vi "Ejemplo7_Strings.vi"() -> ()   [LabVIEW 2020]
panel:
  out "ACTUADOR 3":string
  out "ACTUADOR 2":string
  out "ACTUADOR 1":string
  in  "Contactor":bool
  in  "Termocupla":dbl(slide) scale=0.0..100.0
  in  "Motor":i16(knob) scale=0.0..60.0
  out "length":i32
  out "Salida":string
  in  "Registrar":bool
  in  "Indique Nombre":string
  in  "Indique Apellido":string
  out "Minusculas":string
  out "Mayusculas":string
  out "Subset":string
  out "String Concatenate":string
  out "N Caracteres":i32
  out "Dato B":string
  in  "Dato A":string
  # "Strings"
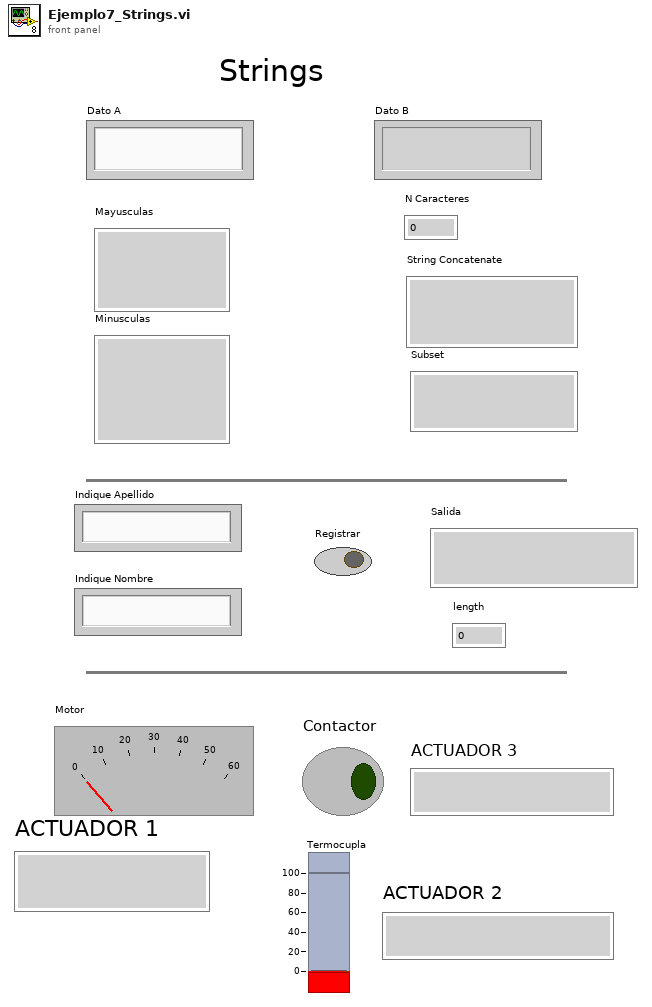
[diagram p1: front panel]
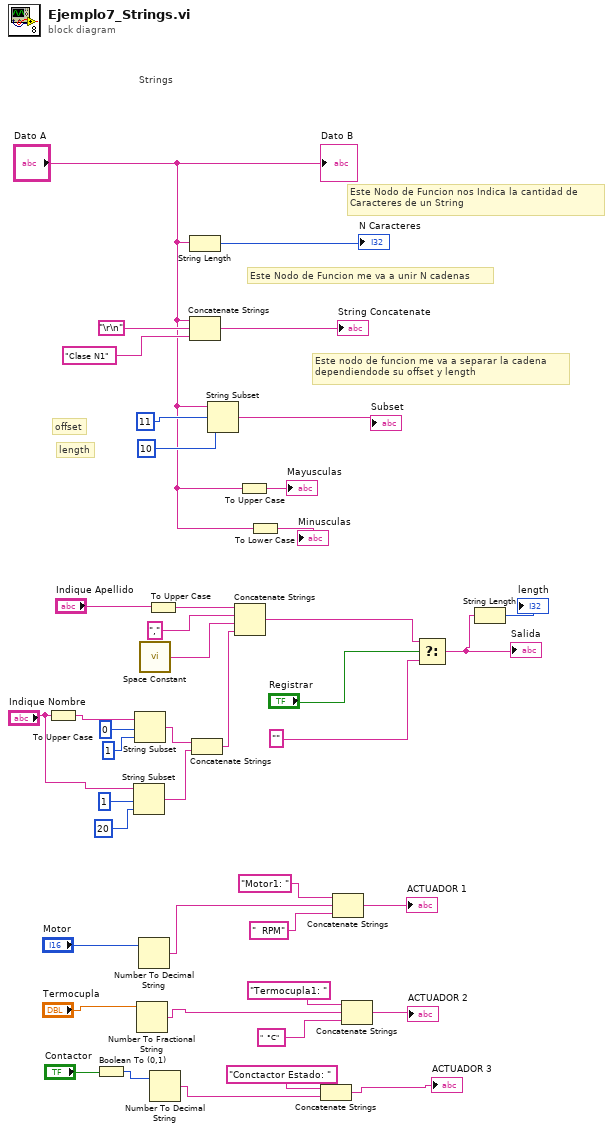
[diagram p0: block diagram]
diagram:
  # "length"
  # "offset"
  # "Este nodo de funcion me va a separar la cadena \ndependiendode su offset y length"
  # "Este Nodo de Funcion me va a unir N cadenas"
  # "Este Nodo de Funcion nos Indica la cantidad de \nCaracteres de un String"
  # "Strings"
  n1 = To Upper Case(1:"Indique Nombre") -> (0:w23:string)
  n2 = Boolean To (0,1)(Boolean="Contactor") -> (0, 1=w4:i16)
  n3 = String Subset(string="Indique Nombre", offset (0)=1 ("length (rest)"), length (rest)=20 ("length (rest)")) -> (substring=w24:string)
  n4 = String Subset(string=w23, offset (0)=0 ("length (rest)"), length (rest)=1 ("length (rest)")) -> (substring=w25:string)
  n5 = Number To Fractional String(number="Termocupla") -> (F-format string=w7:string)  [unwired: 3 in]
  n6 = Number To Decimal String(number="Motor") -> (decimal integer string=w13:string)  [unwired: 1 in]
  n7 = call <vilib>:"Space Constant.vi"() -> ("String"=w30:string)
  n8 = To Upper Case(1:"Indique Apellido") -> (0:w32:string)
  n9 = Number To Decimal String(number=w4) -> (decimal integer string=w2:string)  [unwired: 1 in]
  n10 = String Length(string="Dato A") -> (length=→"N Caracteres":i32)
  n11 = Concatenate Strings("Dato A", "\r\n", "Clase N1") -> (→"String Concatenate":string)
  n12 = Concatenate Strings(w25, w24) -> (w22:string)
  n13 = String Subset(string="Dato A", offset (0)=11, length (rest)=10 ("length (rest)")) -> (substring=→"Subset":string)
  n14 = Concatenate Strings(w32, ",", w30, w22) -> (w20:string)
  n15 = To Upper Case(1:"Dato A") -> (0:→"Mayusculas":string)
  n16 = To Lower Case(string="Dato A") -> (all lower case string=→"Minusculas":string)
  n17 = Concatenate Strings("Conctactor Estado: ", w2) -> (→"ACTUADOR 3":string)
  n18 = Concatenate Strings("Motor1: ", w13, "  RPM") -> (→"ACTUADOR 1":string)
  n19 = Concatenate Strings("Termocupla1: ", w7, "  °C") -> (→"ACTUADOR 2":string)
  n20 = Select(t=w20, s="Registrar", f="") -> (s? t:f=w18:string)
  "Salida" <- w18
  n21 = String Length(string=w18) -> (length=→"length":i32)
  "Dato B" <- "Dato A"
